vi "WriteFloatStringToSerial.vi"() -> ()   [LabVIEW 2017]
uses:
  <vilib>/Instr/_visa.llb/VISA Configure Serial Port (Instr).vi
panel:
  out "Display":string
  in  "Arduino Port":refnum<visa-resource-name>
  in  "Stop Button":bool
  in  "Blink period":dbl=123.45 format="%.2f"
  in  "Write":bool
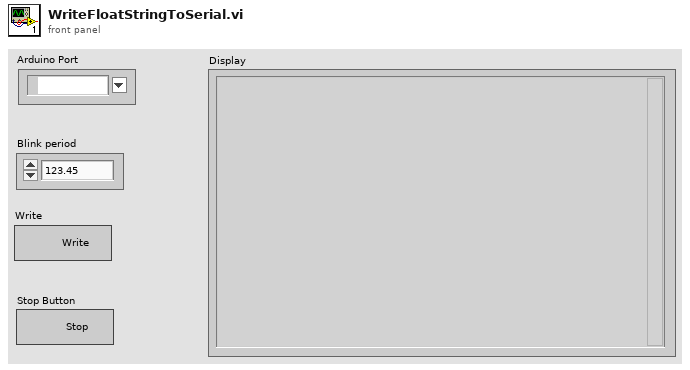
[diagram p1: front panel]
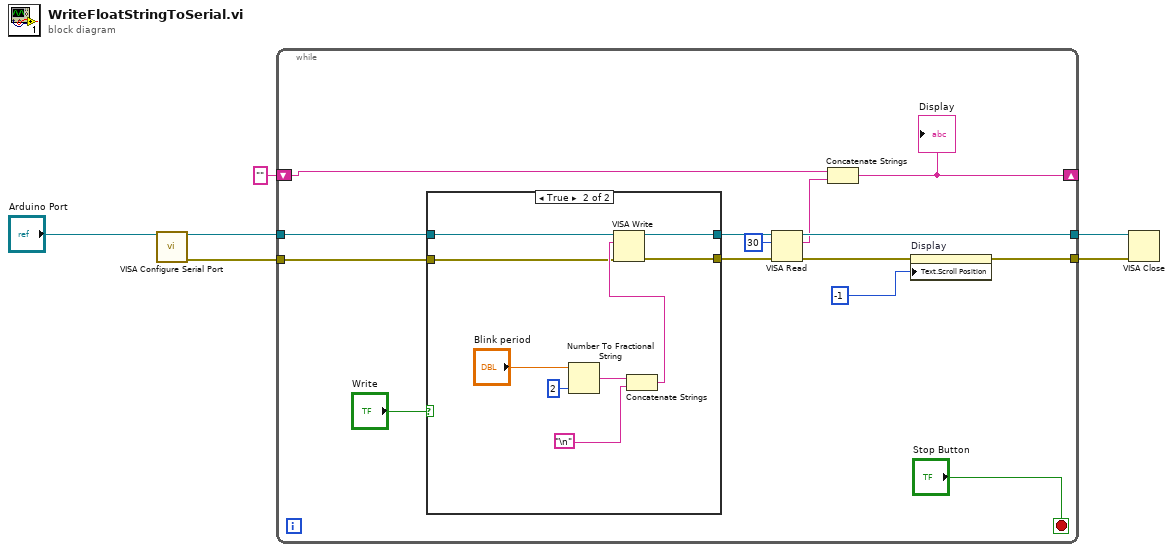
[diagram p0: block diagram]
diagram:
  n1 = call-poly "VISA Configure Serial Port"("VISA resource name"="Arduino Port") -> ("VISA resource name out"=w6:refnum<visa-resource-name>, "error out"=w4:errorcluster)  [unwired: 13 in]
  n2 = while {
    tunnel: w6 -> [w19]
    tunnel: [w17] -> w5
    tunnel: w4 -> [w16]
    tunnel: [w7] -> w3
    shift-right: [w12] -> _
    shift-left: "" -> [w11]
    stop <- "Stop Button" stop-if-true
    n3 = case shown="True" "Write" {
      tunnel: w19 -> [w22 w31]
      tunnel: [w22 w30] -> w18
      tunnel: w16 -> [w21 w25]
      tunnel: [w21 w24] -> w15
      frame False {
      }
      frame True {
        n4 = Number To Fractional String(number="Blink period", precision (6)=i16 2) -> (F-format string=w27:string)  [unwired: 2 in]
        n5 = Concatenate Strings(w27, "\n") -> (w26:string)
        n6 = VISA Write(VISA resource name=w31, write buffer=w26, error in (no error)=w25) -> (VISA resource name out=w30:refnum<visa-resource-name>, error out=w24:errorcluster)  [unwired: 1 out]
      }
    }
    n7 = VISA Read(VISA resource name=w18, byte count=u32 30, error in (no error)=w15) -> (VISA resource name out=w17:refnum<visa-resource-name>, read buffer=w13:string, error out=w8:errorcluster)  [unwired: 1 out]
    n8 = Concatenate Strings(w11, w13) -> (w12:string)
    "Display" <- w12
    n9 = property on="Display" class="Str"(error in=w8, "Text.Scroll Position"=-1) -> (error out=w7:errorcluster)  [unwired: 1 in, 1 out]
  }
  n10 = VISA Close(VISA resource name=w5, error in (no error)=w3) -> ()  [unwired: 1 out]
